vi "Format ROI data cluster.vi"(11 "Single ROI info":dbl[](array[numeric])) -> (3 "X-Y-Z coordinates":T1 {"ROI group ID" format="%#_6f"; "Laser Power (%)" format="%#_6f"; "Zoom" format="%#_6f"; "Frame Size" format="%#_6f"; "Number of lines" format="%#_6f"; "Composite ID" format="%#_6f"; "Angle (deg)" format="%#_6f"; "ROI Time (ns)" format="%#_6f"; "ROI ID" format="%#_6f"; "Pixels in ROI" format="%#_6f"; "ROI index" format="%#_6f"; "Z stop" format="%#_6f"; "Y stop" format="%#_6f"; "X stop" format="%#_6f"; "Z start" format="%#_6f"; "X start" format="%#_6f"; "Y start" format="%#_6f"})   [LabVIEW 2017]
uses:
  Typedefs/ROI parameters data type.ctl
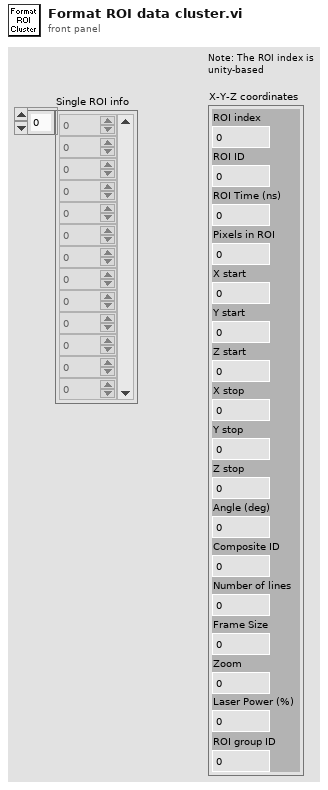
[diagram p1: front panel]
types:
  T1 = typedef "ROI parameters data type.ctl" = cluster{"ROI index":dbl, "ROI ID":dbl, "ROI Time (ns)":dbl, "Pixels in ROI":dbl, "X start":dbl, "Y start":dbl, "Z start":dbl, "X stop":dbl, "Y stop":dbl, "Z stop":dbl, "Angle (deg)":dbl, "Composite ID":dbl, "Number of lines":dbl, "Frame Size":dbl, "Zoom":dbl, "Laser Power (%)":dbl, "ROI group ID":dbl}
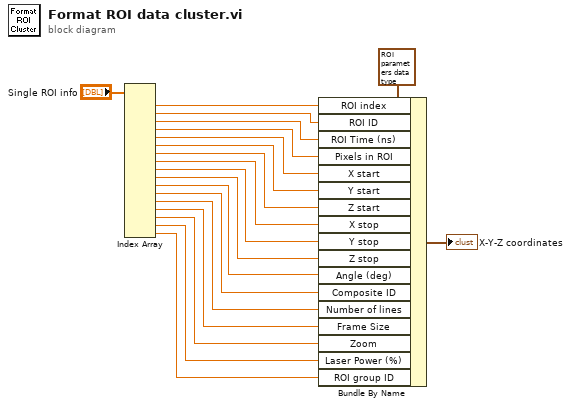
[diagram p0: block diagram]
diagram:
  n1 = Index Array(array="Single ROI info") -> (element #1=w17:dbl, element #2=w16:dbl, element #3=w15:dbl, element #4=w14:dbl, element #5=w13:dbl, element #6=w12:dbl, element #7=w11:dbl, element #8=w10:dbl, element #9=w9:dbl, element #10=w8:dbl, element #11=w7:dbl, element #12=w6:dbl, element #13=w5:dbl, element #14=w4:dbl, element #15=w3:dbl, element #16=w2:dbl, element #17=w1:dbl)  [unwired: 17 in]
  n2 = Bundle By Name(cluster=T1 {"ROI index"=0.0, "ROI ID"=0.0, "ROI Time (ns)"=0.0, "Pixels in ROI"=0.0, "X start"=0.0, "Y start"=0.0, "Z start"=0.0, "X stop"=0.0, "Y stop"=0.0, "Z stop"=0.0, "Angle (deg)"=0.0, "Composite ID"=0.0, "Number of lines"=0.0, "Frame Size"=0.0, "Zoom"=0.0, "Laser Power (%)"=0.0, "ROI group ID"=0.0} ("X-Y-Z coordinates"), "ROI index"=w17, "ROI ID"=w16, "ROI Time (ns)"=w15, "Pixels in ROI"=w14, "X start"=w13, "Y start"=w12, "Z start"=w11, "X stop"=w10, "Y stop"=w9, "Z stop"=w8, "Angle (deg)"=w7, "Composite ID"=w6, "Number of lines"=w5, "Frame Size"=w4, "Zoom"=w3, "Laser Power (%)"=w2, "ROI group ID"=w1) -> (→"X-Y-Z coordinates":T1)
